vi "APP_FGV_ApplicationEvtCmfRef.vi"(8 "error in":errorcluster) -> (0 "error out":errorcluster, 3 "App_Evt":refnum<user-event>)   [LabVIEW 2012, in "APP_AppControl.lvlib"]
uses:
  APP_AppControl.lvlib
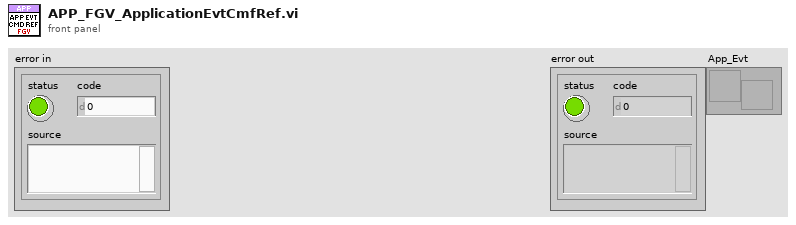
[diagram p1: front panel]
types:
  T1 = cluster{"App_EvtCmds":enum16{"CLOSE_APP"}, "variant":variant}
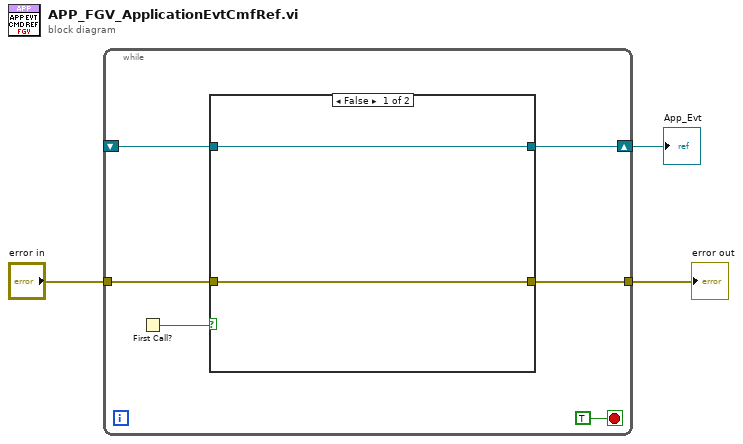
[diagram p0: block diagram]
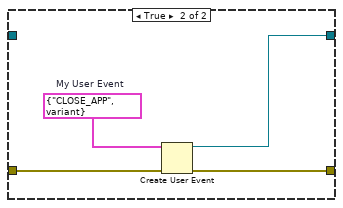
[diagram p2: hidden frame]
diagram:
  n1 = while {
    tunnel: "error in" -> [w7]
    tunnel: [w6] -> w2
    shift-right: [w5] -> w1
    shift-left: _ -> [w4]
    stop <- TRUE stop-if-true
    n2 = First Call?() -> (First Call?: T/F=w8:bool)
    n3 = case shown="False" w8 {
      tunnel: w7 -> [w10 w15]
      tunnel: [w10 w14] -> w6
      tunnel: [w11 w12] -> w5
      tunnel: w4 -> [w11 _]
      frame False {
      }
      frame True {
        w13 = T1 {"App_EvtCmds"=enum."CLOSE_APP", "variant"=variant}  # My User Event
        n4 = Create User Event(user event datatype=w13, error in=w15) -> (user event=w12:refnum<user-event>, error out=w14:errorcluster)
      }
    }
  }
  "error out" <- w2
  "App_Evt" <- w1
